vi "Create.vi"(8 "error in (no error)":errorcluster, 10 "ID tag":string, 11 "Instrument in":refnum<class "Instrument.lvclass">) -> (0 "error out":errorcluster, 3 "InstrPtr out":refnum<class "InstrPtr.lvclass">)   [LabVIEW 2009, in "InstrPtr.lvclass"]
doc: "The Instrument Pointer Class allows access to Instrument objects on the heap instead of on the stack. It accesses them in a thread-safe manner by using an internal reference queue. In other words, multiple programs can share the same Instrument class and read/write to the same variables, which keeps all references to the Instrument in sync with one another.\n\nSee LabVIEW\\examples\\lvoop\\ReferenceObject for details.\n\nDereference: this \"checks out\" the object, which you can then mutate with the standard accessor methods for the class. All other programs will wait (block) on this method until you check the object back in.\n\nReference: this \"checks in\" the object when you are done with it. Other classes will wait (block) to use the instrument until you check it back in."
uses:
  InstrPtr.lvclass
  Instrument/Instrument.lvclass
  InstrPtr.lvclass/InstrPtr.ctl
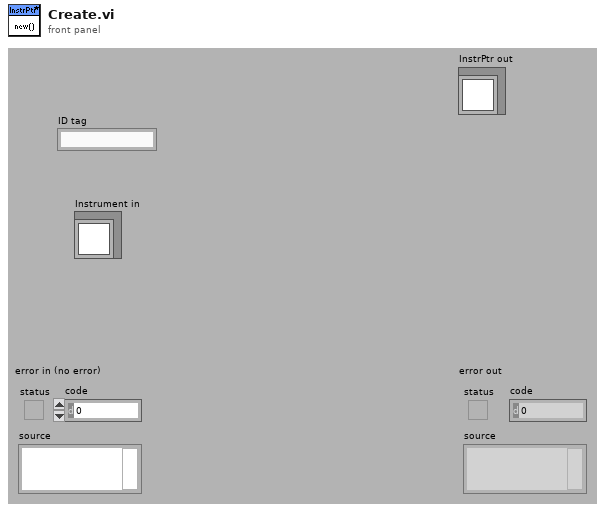
[diagram p1: front panel]
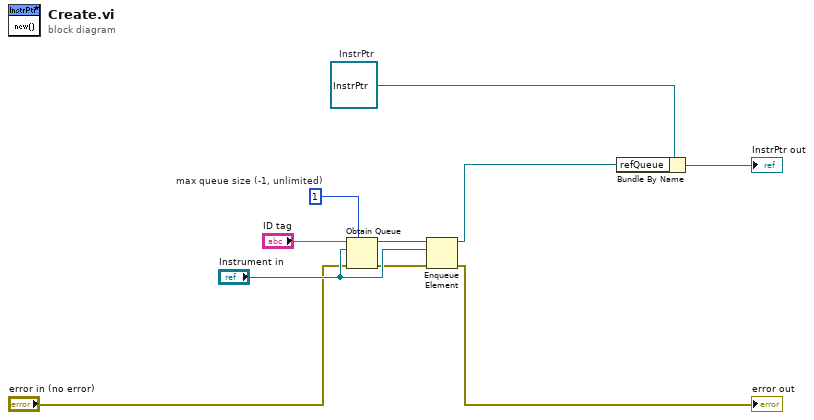
[diagram p0: block diagram]
diagram:
  w1 = 1  # max queue size (-1, unlimited)
  w8 = refnum<class "InstrPtr.lvclass"> refnum  # InstrPtr
  n1 = Obtain Queue(max queue size (-1, unlimited)=w1, name (unnamed)="ID tag", element data type="Instrument in", error in (no error)="error in (no error)") -> (queue out=w7:refnum<queue>, error out=w2:errorcluster)  [unwired: 1 in, 1 out]
  n2 = Enqueue Element(queue=w7, element="Instrument in", error in (no error)=w2) -> (queue out=w6:refnum<queue>, error out=→"error out":errorcluster)  [unwired: 2 out]
  n3 = Bundle By Name(cluster=w8, "refQueue"=w6) -> (→"InstrPtr out":refnum<class "InstrPtr.lvclass">)
